vi "Untitled 1.vi"() -> ()   [LabVIEW 2026]
uses:
  <vilib>/Instr/_visa.llb/VISA Configure Serial Port (Instr).vi
panel:
  in  "打开串口":bool
  out "串口打开状态":bool
  in  "stop bits (10: 1 bit)":u16(ring)=10 items=["1.0"=10, "1.5"=15, "2.0"=20]
  in  "parity (0:none)":enum16{"None", "Odd", "Even", "Mark", "Space"}(ring)
  in  "data bits (8)":u16=8 min=5 max=8 step=1
  in  "baud rate (9600)":u32=9600
  in  "VISA resource name":refnum<visa-resource-name>
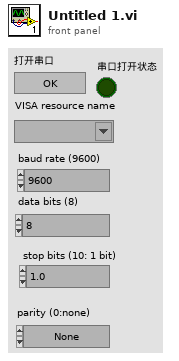
[diagram p1: front panel]
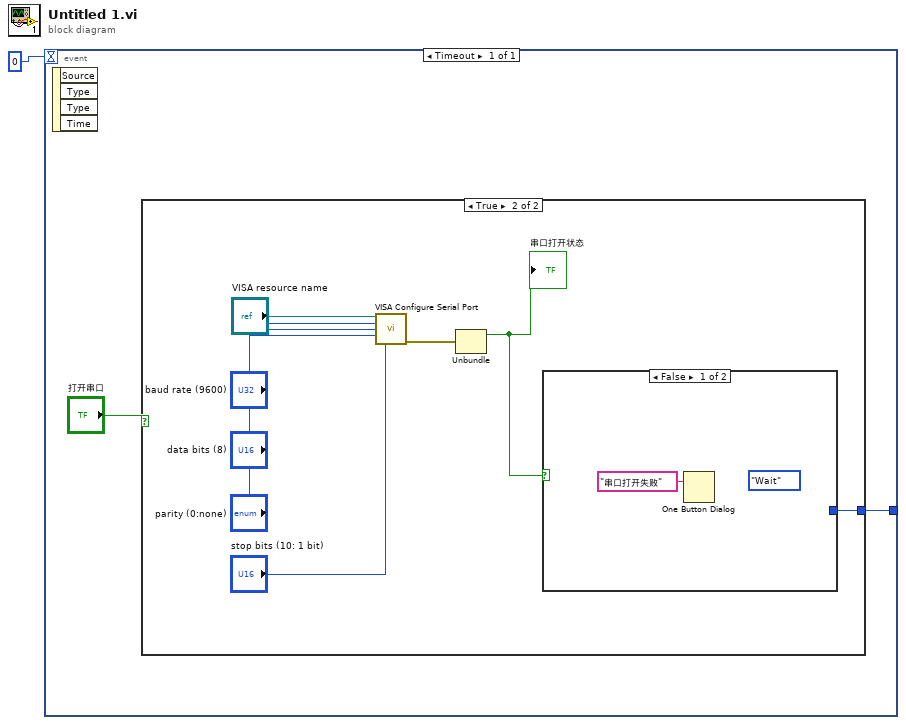
[diagram p0: block diagram]
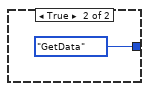
[diagram p3: hidden frame]
diagram:
  n1 = event shown="[0] Timeout" {
    selector: _ -> [_]
    dyn-events: _ -> [_]
    timeout: 0 -> [_]
    tunnel: [w2] -> _
    event Timeout {
      n2 = event-data() -> ()  [unwired: 1 in, 4 out]
      n3 = case shown="True" "打开串口" {
        tunnel: [_ w4] -> w2
        frame False {
        }
        frame True {
          n4 = call-poly "VISA Configure Serial Port"("VISA resource name"="VISA resource name", "baud rate (9600)"="baud rate (9600)", "data bits (8)"="data bits (8)", "parity (0:none)"="parity (0:none)", "stop bits (10: 1 bit)"="stop bits (10: 1 bit)") -> ("error out"=w6:errorcluster)  [unwired: 9 in, 1 out]
          n5 = Unbundle(w6) -> ("status"=w5:bool)  [unwired: 2 out]
          "串口打开状态" <- w5
          n6 = case shown="False" w5 {
            tunnel: [_ enum16{"GetData"}."GetData"] -> w4
            frame False {
              (unwired) enum16{"Wait"}."Wait"
              n7 = One Button Dialog(message="串口打开失败") -> ()  [unwired: 1 in, 1 out]
            }
            frame True {
            }
          }
        }
      }
    }
  }
